vi "Parse Sheet to JSON.vi"(7 "SpreadsheetDocument in":refnum<k24>, 8 "error in":errorcluster, 9 "Cells":cluster{"Cells":variant[][]}[](array[cluster]), 10 "Named Ranges":string[](array[string]), 11 "<JSON> in":string) -> (0 "error out":errorcluster, 3 "<JSON> out":string)   [LabVIEW 2025, in "Config from EXCEL.lvclass"]
uses:
  Config from EXCEL.lvclass
  Config from EXCEL.lvclass/Config from EXCEL.ctl
  <vilib>/JDP Science/JSONtext/JSONtext.lvlib
  D:/git/Open-Xml-LabVIEW/dll/DocumentFormat.OpenXml.dll
  Open-Xml-LabVIEW/dll/DocumentFormat.OpenXml.dll
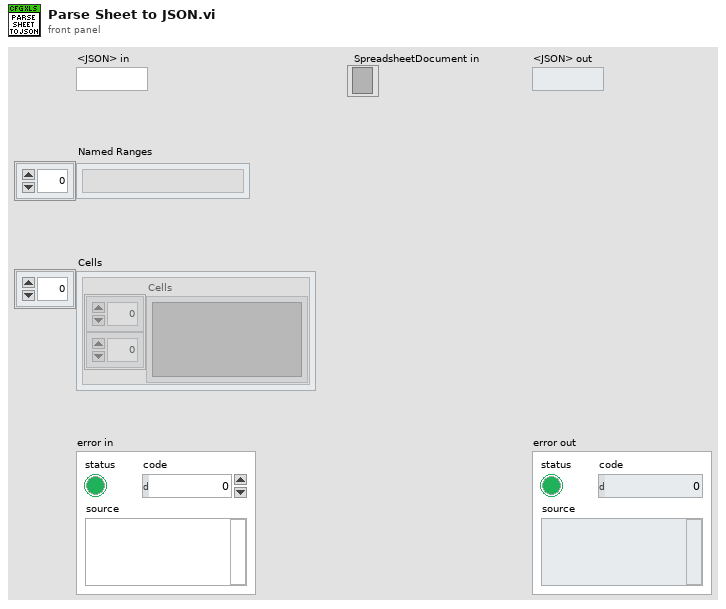
[diagram p1: front panel]
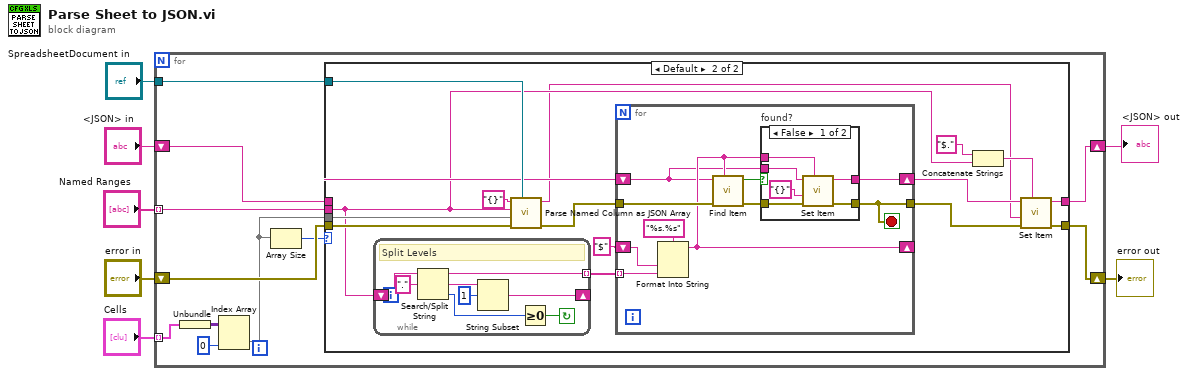
[diagram p0: block diagram]
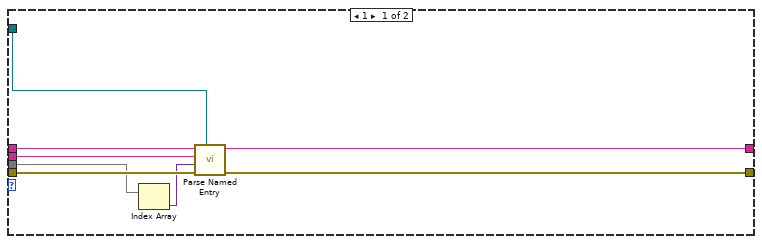
[diagram p2: hidden frame]
diagram:
  n1 = for {
    shift-right: [w13] -> w6
    shift-left: "error in" -> [w16]
    shift-right: [w14] -> w7
    shift-left: "<JSON> in" -> [w17]
    tunnel: "Named Ranges" -> [w12] mode=indexing
    tunnel: "Cells" -> [w9] mode=indexing
    tunnel: "SpreadsheetDocument in" -> [w15]
    n2 = Unbundle(w9) -> ("Cells"=w8:variant[][])
    n3 = Index Array(array=w8, index (col)=0) -> (element=w11:variant[])  [unwired: 1 in]
    n4 = Array Size(array=w11) -> (size(s)=w10:i32)
    n5 = case shown="1" w10 {
      tunnel: w17 -> [w24 w35]
      tunnel: w16 -> [w25 w42]
      tunnel: w15 -> [w19 w41]
      tunnel: [w23 w27] -> w14
      tunnel: [w26 w29] -> w13
      tunnel: w12 -> [w22 w33]
      tunnel: w11 -> [w21 w40]
      frame 1 {
        n6 = Index Array(array=w21) -> (element=w20:variant)  [unwired: 1 in]
        n7 = call "Parse Named Entry.vi"("SpreadsheetDocument in"=w19, "error in"=w25, "Cells"=w20, "Named Range"=w22, "<JSON>"=w24) -> ("error out"=w26:errorcluster, "<JSON> out"=w23:string)  [unwired: 5 in]
      }
      frame Default {
        n8 = while {
          shift-right: [w63] -> _
          shift-left: w33 -> [w62]
          tunnel: [w61] -> w37 mode=indexing
          stop <- w64 continue-if-true
          # "Split Levels"
          n9 = Search/Split String(string=w62, search string/char (-)=".") -> (substring before match=w61:string, match + rest of string=w65:string, offset of match=w67:i32)  [unwired: 1 in]
          n10 = String Subset(string=w65, offset (0)=1) -> (substring=w63:string)  [unwired: 1 in]
          n11 = Greater Or Equal To 0?(x=w67) -> (x >= 0?=w64:bool)
        }
        n12 = call "Parse Named Column as JSON Array.vi"("SpreadsheetDocument in"=w41, "error in"=w42, "Cells"=w40, "Named Range"=w33, "<JSON>"="{}") -> ("error out"=w38:errorcluster, "<JSON> out"=w28:string)  [unwired: 5 in]
        n13 = for {
          tunnel: w37 -> [w50] mode=indexing
          shift-right: [w45] -> _
          shift-left: "$" -> [w51]
          tunnel: w38 -> [w48]
          tunnel: [w47] -> w31
          shift-right: [w44] -> w30
          shift-left: w35 -> [w43]
          stop <- w47 stop-if-true
          n14 = Format Into String(format string="%s.%s", w51, w50) -> (resulting string=w45:string)  [unwired: 2 in, 1 out]
          n15 = call <vilib>:"Find Item.vi"("$Path or Item Name"=w45, "error in (no error)"=w48, "JSON"=w43) -> ("error out"=w49:errorcluster, "Found"=w46:bool)  [unwired: 5 in, 2 out]
          n16 = case "found?" shown="False" w46 {
            tunnel: [w57 w59] -> w44
            tunnel: [w56 w60] -> w47
            tunnel: w49 -> [w55 w60]
            tunnel: w45 -> [w54 _]
            tunnel: w43 -> [w53 w59]
            frame False {
              n17 = call <vilib>:"Set Item.vi"("$Path or Item Name"=w54, "error in (no error)"=w55, "JSON to Insert"="{}", "JSON"=w53) -> ("error out"=w56:errorcluster, "<JSON>"=w57:string)  [unwired: 4 in, 1 out]
            }
            frame True {
            }
          }
        }
        n18 = Concatenate Strings("$." ("string"), w33) -> (w32:string)
        n19 = call <vilib>:"Set Item.vi"("$Path or Item Name"=w32, "error in (no error)"=w31, "JSON to Insert"=w28, "JSON"=w30) -> ("error out"=w29:errorcluster, "<JSON>"=w27:string)  [unwired: 4 in, 1 out]
      }
    }
  }
  "<JSON> out" <- w7
  "error out" <- w6
